vi "sv_Resample Engine (Time to Angle).vi"(5 "reset? (True)":bool=TRUE, 8 "error in (no error)":errorcluster, 9 "filter prototype":T2={"left wing"=[], "increment"=[], "max dec"=128, "timing jitter"=enum."Interpolation", "band limiting?"=TRUE} {"increment" format="%.2f"; "left wing" format="%.2f"}, 10 "time":dbl[](array[numeric]) format="%.2f", 11 "scaled signals (EU)":waveform(dbl)[](array[waveform])) -> (0 "error out":errorcluster, 1 "offset":dbl, 2 "time stamps":dbl[](array[numeric]) format="%.2f", 3 "Y":dbl[][](array[numeric]) format="%.2f")   [LabVIEW 2017, in "SoundVib_ContSweptSine.lvlib"]
doc: "Perform an arbitrary resampling on the input signal."
uses:
  <vilib>/addons/Sound and Vibration/svt_Continuous Swept Sine/SoundVib_ContSweptSine.lvlib
  <vilib>/addons/_NISVFA/_Shared subVIs/Controls/OAT Resample Filter Prototype.ctl
  <vilib>/addons/Sound and Vibration/Order Analysis/Resample Order Tracking/SoundVib_Resampling.lvlib
  <resource>/sndvib.dll
panel:
  in  "state in":T1 {"time interval" format="%.2f"; "position" format="%.2f"; "init condition" format="%.2f"}
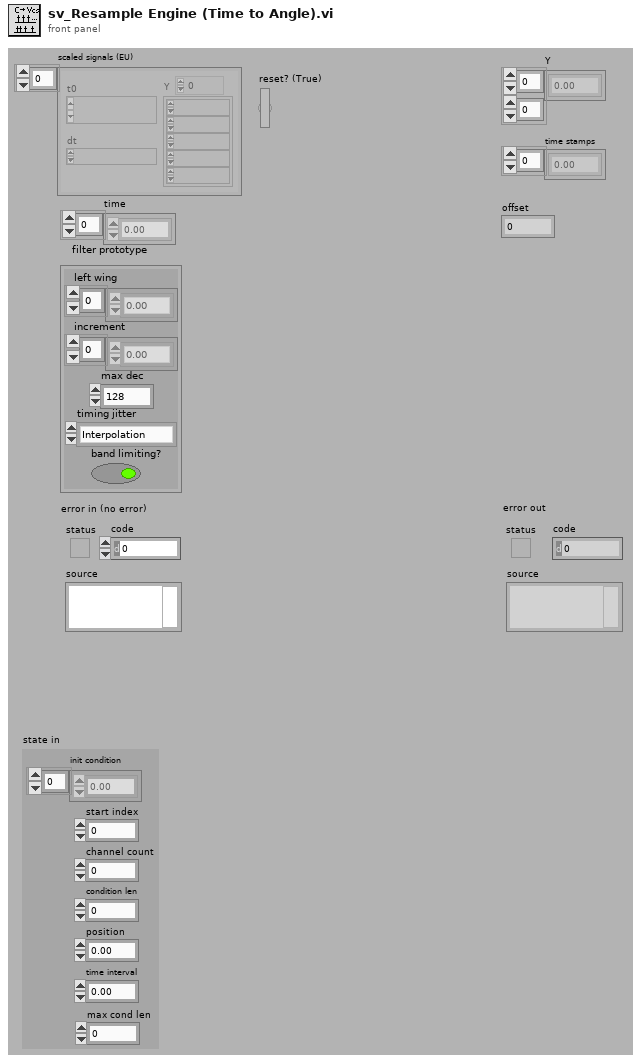
[diagram p1: front panel]
types:
  T1 = cluster{"init condition":dbl[], "start index":i32, "channel count":i32, "condition len":i32, "position":dbl, "time interval":dbl, "max cond len":i32}
  T2 = typedef "OAT Resample Filter Prototype.ctl" = cluster{"left wing":dbl[], "increment":dbl[], "max dec":i32, "timing jitter":enum32{"Interpolation", "Rounding"}, "band limiting?":bool}
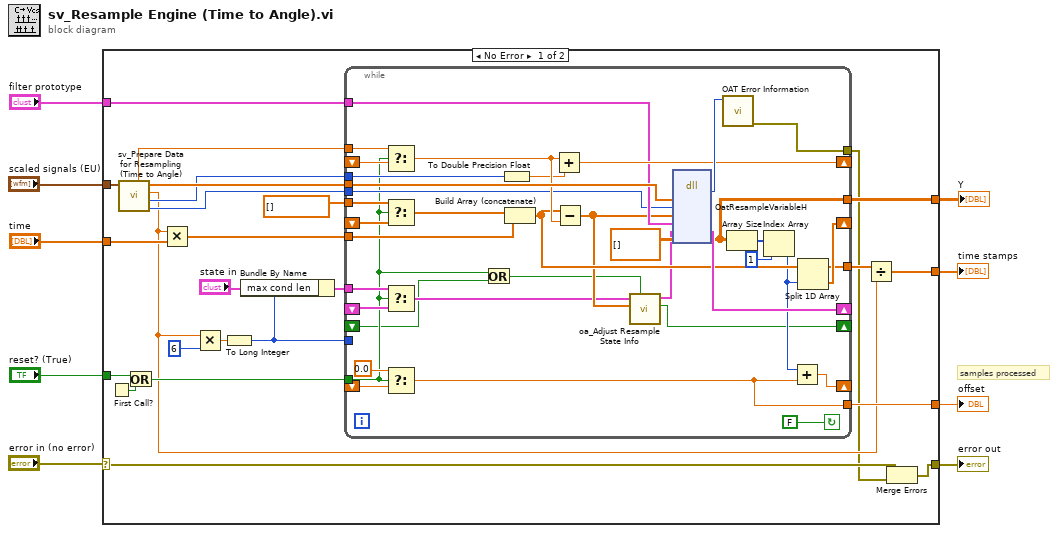
[diagram p0: block diagram]
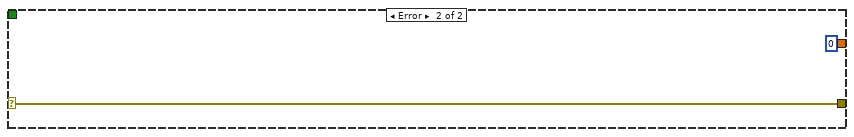
[diagram p2: hidden frame]
diagram:
  # "samples processed"
  n1 = case shown="No Error" "error in (no error)" {
    selector: "error in (no error)" -> [w13 w74]
    tunnel: "filter prototype" -> [w34 _]
    tunnel: "time" -> [w33 _]
    tunnel: [w30 _] -> w7
    tunnel: [w28 0] -> w6
    tunnel: [w11 w74] -> w5
    tunnel: "scaled signals (EU)" -> [w31 _]
    tunnel: [w24 _] -> w2
    tunnel: "reset? (True)" -> [w21 _]
    frame No Error {
      n2 = First Call?() -> (First Call?: T/F=w22:bool)
      n3 = call <vilib>:"sv_Prepare Data for Resampling (Time to Angle).vi"("Array"=w31) -> ("channel count"=w25:i32, "signal len"=w27:i32, "fs"=w19:dbl, "Y"=w32:dbl[], "elapsed length"=w10:dbl)  [unwired: 6 in]
      n4 = Or(x=w21, y=w22) -> (x .or. y?=w20:bool)
      n5 = Multiply(x=w19, y=w33) -> (x*y=w23:dbl[])
      n6 = Multiply(x=w19, y=6) -> (x*y=w17:dbl)
      n7 = To Long Integer(number=w17) -> (32bit integer=w15:i32)
      n8 = Bundle By Name(cluster="state in", "max cond len"=w15) -> (w14:T1)
      n9 = while {
        shift-right: [w53] -> _
        shift-left: _ -> [w65]
        tunnel: w32 -> [w68]
        tunnel: w23 -> [w67]
        shift-right: [w63] -> _
        shift-left: _ -> [w69]
        tunnel: w20 -> [w37]
        tunnel: w34 -> [w54]
        shift-right: [w59] -> _
        shift-left: _ -> [w61]
        tunnel: [w70] -> w12
        tunnel: [w40] -> w30
        tunnel: w14 -> [w66]
        tunnel: dbl[] [] ("t") -> [w62]
        tunnel: [w51] -> w26
        tunnel: [w57] -> w28
        shift-right: [w55] -> _
        shift-left: _ -> [w58]
        tunnel: w27 -> [w50]
        tunnel: w25 -> [w52]
        tunnel: w15 -> [_]
        tunnel: w10 -> [w39]
        shift-right: [w38] -> _
        shift-left: _ -> [w36]
        stop <- FALSE continue-if-true
        n10 = Select(t=w39, s=w37, f=w58) -> (s? t:f=w56:dbl)
        n11 = Select(t=w62, s=w37, f=w69) -> (s? t:f=w64:dbl[])
        n12 = Select(t=w66, s=w37, f=w65) -> (s? t:f=w42:T1)
        n13 = Select(t=0.0, s=w37, f=w61) -> (s? t:f=w57:dbl)
        n14 = Or(x=w37, y=w36) -> (x .or. y?=w35:bool)
        n15 = To Double Precision Float(number=w50) -> (double precision float=w49:dbl)
        n16 = Build Array (concatenate)(w64, w67) -> (w48:dbl[])
        n17 = Add(x=w56, y=w49) -> (x+y=w55:dbl)
        n18 = Subtract(x=w48, y=w56) -> (x-y=w43:dbl[])
        n19 = call <vilib>:"oa_Adjust Resample State Info.vi"("Reset? (True)"=w35, "time position"=w43, "state in"=w42) -> ("reset pending"=w38:bool, "state out"=w41:T1)  [unwired: 7 in]
        n20 = dll-call lib="C:/Program Files (x86)/National Instruments/LabVIEW 2017/resource/sndvib.*" fn="OatResampleVariableH"("signalH"=w68, "channelCount"=w52, "timeH"=w43, "prototype"=w54, "state"=w41, "yH"=dbl[][] []) -> ("return type"=w71:i32, "state"=w53:T1, "yH"=w40:dbl[][])  [unwired: 7 in, 2 out]
        n21 = call <vilib>:"OAT Error Information.vi"("error code"=w71) -> ("error out"=w70:errorcluster)  [unwired: 6 in]
        n22 = Array Size(array=w40) -> (size(s)=w46:i32[])
        n23 = Index Array(array=w46, index=1) -> (element=w44:i32)
        n24 = Add(x=w44, y=w57) -> (x+y=w59:dbl)
        n25 = Split 1D Array(array=w48, index=w44) -> (first subarray=w51:dbl[], second subarray=w63:dbl[])
      }
      n26 = Divide(x=w26, y=w19) -> (x/y=w24:dbl[])
      n27 = Merge Errors(w13, w12) -> (w11:errorcluster)
    }
    frame Error {
    }
  }
  "time stamps" <- w2
  "Y" <- w7
  "offset" <- w6
  "error out" <- w5
